vi "CreateStatedetHDF5.vi"(5 "det_hardware":enum16{"CAMERA", "PMT"}(ring), 7 "attributes":T1, 8 "error in (no error)":errorcluster, 9 "PMT readout":i16[][](array[numeric]), 10 "kinetic series data":i16[][][][](array[numeric]), 11 "appended path":path) -> (0 "error out":errorcluster)   [LabVIEW 2019]
uses:
  <vilib>/Utility/miscctls.llb/LVRectTypeDef.ctl
  <vilib>/UPVI/lvhdf5/group.llb/H5G_obj_t.ctl
  <vilib>/UPVI/lvhdf5/dataset.llb/LVH5D Operation.ctl
  <vilib>/UPVI/lvhdf5/group.llb/OpenCreateGroup (String).vi
  <vilib>/Utility/VariantDataType/GetClusterInfo.vi
  <vilib>/Utility/VariantDataType/GetTypeInfo.vi
  <vilib>/UPVI/lvhdf5/attribute.llb/Write Multiple Attributes.vi
  <vilib>/UPVI/lvhdf5/utility.llb/Select HDF5 Dialog.vi
  <vilib>/UPVI/lvhdf5/utility.llb/Select HDF5 Dialog (Object Only).vi
  <vilib>/UPVI/lvhdf5/dataset.llb/Simple H5Dwrite (Variant).vi
  <vilib>/UPVI/lvhdf5/attribute.llb/LVH5A Operation.ctl
  <vilib>/UPVI/lvhdf5/attribute.llb/LVH5 Write Attributes.xnode
  <vilib>/UPVI/lvhdf5/library.llb/HDF5 Ref.ctl
  <vilib>/UPVI/lvhdf5/attribute.llb/Cluster to Attribute Array.xnode
  <vilib>/UPVI/lvhdf5/dataset.llb/Simple H5Dwrite.xnode
  <vilib>/Utility/VariantDataType/VariantType.lvlib
  <vilib>/UPVI/lvhdf5/identifier.llb/Not an HDF5 Refnum Constant.vi
  <vilib>/Utility/error.llb/Error Cluster From Error Code.vi
  <vilib>/UPVI/lvhdf5/dataset.llb/OpenCreateReplace Dataset by Element Type.vi
  <vilib>/UPVI/lvhdf5/dataspace.llb/H5Sselect_hyperslab.vi
  <vilib>/UPVI/lvhdf5/dataset.llb/H5Dwrite (Variant).vi
  <vilib>/UPVI/lvhdf5/dataset.llb/H5Dget_space.vi
  <vilib>/UPVI/lvhdf5/attribute.llb/private/LVH5AwriteWDTAttrs.vi
  <vilib>/UPVI/lvhdf5/dataspace.llb/H5Sclose.vi
  <vilib>/UPVI/lvhdf5/dataset.llb/H5Dclose.vi
  <vilib>/UPVI/lvhdf5/file.llb/OpenCreateReplace HDF5 File.vi
  <vilib>/UPVI/lvhdf5/file.llb/LVH5F Operation.ctl
  <vilib>/UPVI/lvhdf5/utility.llb/Select HDF5 Dialog (File and Object).vi
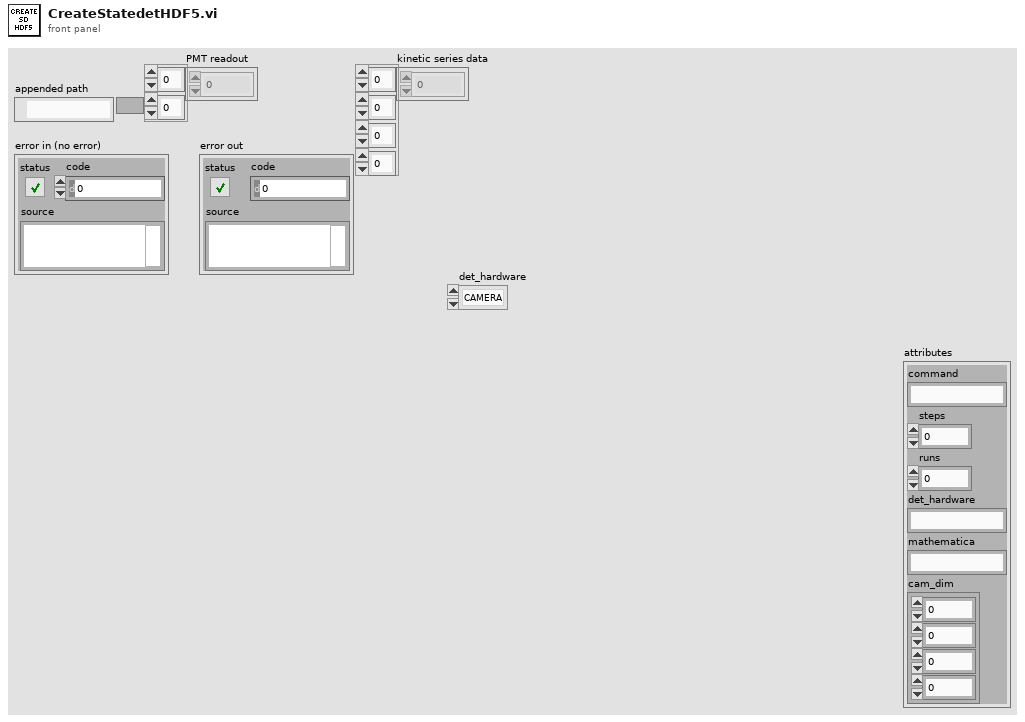
[diagram p1: front panel]
types:
  T1 = cluster{"command":string, "steps":dbl, "runs":dbl, "det_hardware":string, "mathematica":string, "cam_dim":cluster{i32, i32, i32, i32}}
  T2 = typedef "HDF5 Ref.ctl" = refnum<k1>
  T3 = typedef "LVRectTypeDef.ctl" = cluster{"Left":i16, "Top":i16, "Right":i16, "Bottom":i16}
  T4 = cluster{"Behavior":enum32{"Invalid", "Default", "Floating", "Floating/Auto-Hide", "Modal"}, "Position":T3, "Center":bool, "Title":string}
  T5 = typedef "LVH5F Operation.ctl" = enum16{"open", "open or create", "create or replace", "create or replace (with confirmation)", "create", "open (read only)"}
  T6 = typedef "LVH5D Operation.ctl" = enum16{"open", "replace", "create", "open or create", "create or replace", "create or replace with confirmation"}
  T7 = typedef "H5G_obj_t.ctl" = i32
  T8 = cluster{"Object Types (any)":T7[], "Object Pattern":string}
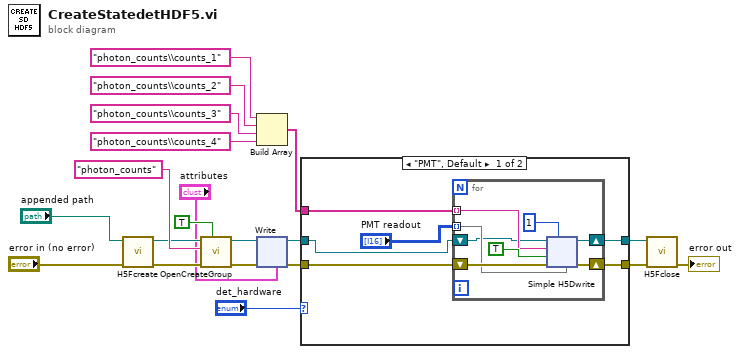
[diagram p0: block diagram]
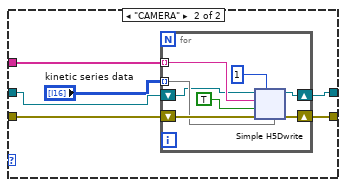
[diagram p2: hidden frame]
diagram:
  n1 = call <vilib>:"H5Fcreate.vi"("error in (no error)"="error in (no error)", "path"="appended path") -> ("error out"=w17:errorcluster, "HDF5 Ref"=w16:T2)  [unwired: 6 in]
  n2 = call-poly <vilib>:"OpenCreateGroup.vi"("Create if not found (F)"=TRUE, "error in (no error)"=w17, "Group"="photon_counts", "HDF5 Ref"=w16) -> ("error out"=w5:errorcluster, "HDF5 Ref out"=w6:T2)  [unwired: 5 in, 1 out]
  n3 = Build Array("photon_counts\\counts_1" ("Dataset Path"), "photon_counts\\counts_2" ("Dataset Path"), "photon_counts\\counts_3" ("Dataset Path"), "photon_counts\\counts_4" ("Dataset Path")) -> (w9:string[])
  n4 = xnode "Write"("HDF5 Ref"=w6, "error in (no error)"=w5, "Value(s)"="attributes") -> ("HDF5 Ref out"=w3:T2, "error out"=w2:errorcluster)  [unwired: 2 in]
  n5 = case shown="\"PMT\", Default" "det_hardware" {
    tunnel: w9 -> [w26 w242]
    tunnel: [w25 w241] -> w8
    tunnel: [w24 w240] -> w7
    tunnel: w3 -> [w23 w239]
    tunnel: w2 -> [w22 w238]
    frame "PMT", Default {
      n6 = for {
        shift-right: [w34] -> w24
        shift-left: w23 -> [w27]
        shift-right: [w32] -> w25
        shift-left: w22 -> [w31]
        tunnel: w26 -> [w28] mode=indexing
        tunnel: "PMT readout" -> [w30] mode=indexing
        n7 = xnode "Simple H5Dwrite"("Compression Level (0-disabled)"=1, "Dataset Path"=w28, "Unlimited  dataset (F)"=TRUE, "error in (no error)"=w31, "HDF5 Path or Ref"=w27, "Data"=w30) -> ("HDF5 Ref out"=w34:T2, "error out"=w32:errorcluster)  [unwired: 2 in, 1 out]
      }
    }
    frame "CAMERA" {
      n8 = for {
        shift-right: [w250] -> w240
        shift-left: w239 -> [w243]
        shift-right: [w248] -> w241
        shift-left: w238 -> [w247]
        tunnel: w242 -> [w244] mode=indexing
        tunnel: "kinetic series data" -> [w246] mode=indexing
        n9 = xnode "Simple H5Dwrite"("Compression Level (0-disabled)"=1, "Dataset Path"=w244, "Unlimited  dataset (F)"=TRUE, "error in (no error)"=w247, "HDF5 Path or Ref"=w243, "Data"=w246) -> ("HDF5 Ref out"=w250:T2, "error out"=w248:errorcluster)  [unwired: 2 in, 1 out]
      }
    }
  }
  n10 = call <vilib>:"H5Fclose.vi"("error in (no error)"=w8, "HDF5 Ref"=w7) -> ("error out"=→"error out":errorcluster)  [unwired: 7 in]
